vi "Watchdog (SubVI).vi"(7 "System Message Queue In":refnum<queue>, 8 "error in (no error)":errorcluster, 11 "Enable Watchdog?":bool) -> (0 "error out":errorcluster)   [LabVIEW 2019]
uses:
  Globals and Definitions/System Message.ctl
  <vilib>/RTwatchdog.llb/Watchdog expiration actions.ctl
  <vilib>/RTwatchdog.llb/Watchdog status enum.ctl
  Globals and Definitions/Initialization Globals.vi
  Globals and Definitions/RT Globals RD v1.0.vi
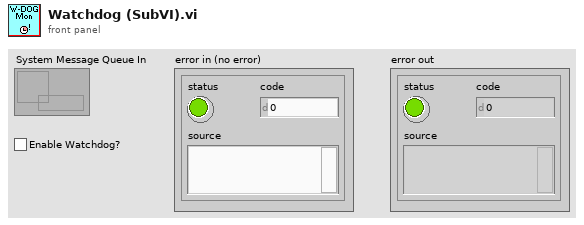
[diagram p1: front panel]
types:
  T1 = typedef "System Message.ctl" = cluster{"Message Tag":string, "Message Body":string, "Snooze Time (s)":dbl, "Snooze Alert?":bool, "Log Event?":bool, "Send Email":i32}
  T2 = typedef "Watchdog expiration actions.ctl" = cluster{"reset system":bool, "restart LabVIEW Runtime":bool, "occurrence":bool, "trigger protocol":enum16{"active high", "active low", "open collector"}, "trigger line":enum16{"none", "line 0", "line 1", "line 2", "line 3", "line 4", "line 5", "line 6", "line 7", "SMB line 0"}, "disable watchdog on VI exit":bool}
  T3 = typedef "Watchdog status enum.ctl" = enum16{"disabled", "expired", "running"}
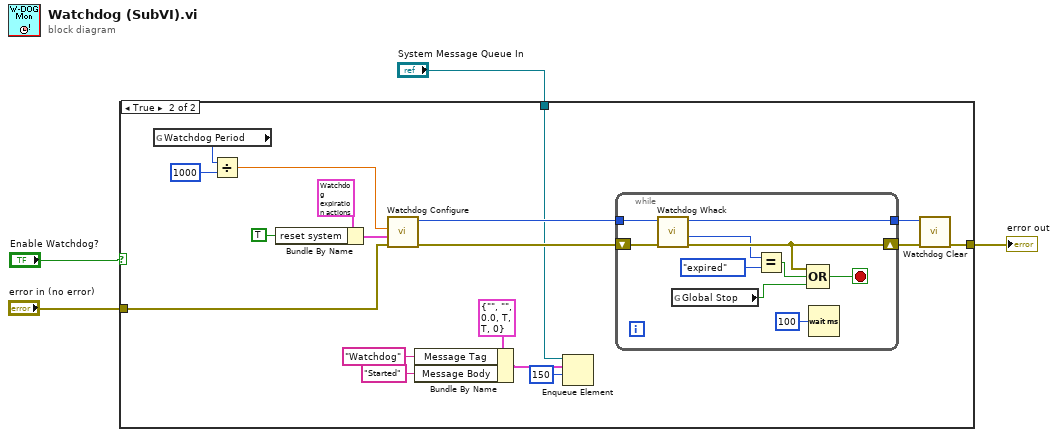
[diagram p0: block diagram]
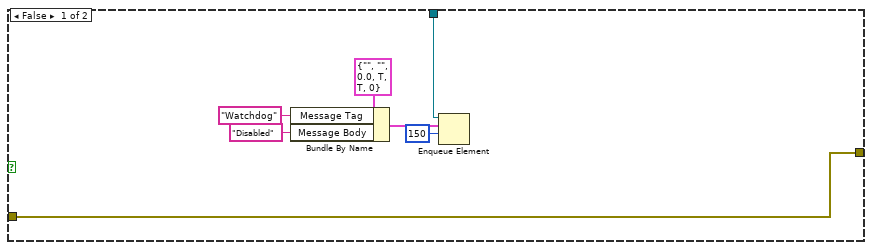
[diagram p2: hidden frame]
diagram:
  n1 = case shown="True" "Enable Watchdog?" {
    tunnel: "error in (no error)" -> [w11 w23]
    tunnel: [w11 w22] -> w2
    tunnel: "System Message Queue In" -> [w6 w15]
    frame False {
      n2 = Bundle By Name(cluster=T1 {"Message Tag"="", "Message Body"="", "Snooze Time (s)"=0.0, "Snooze Alert?"=TRUE, "Log Event?"=TRUE, "Send Email"=0}, "Message Tag"="Watchdog", "Message Body"="Disabled") -> (w5:T1)
      n3 = Enqueue Element(queue=w6, element=w5, timeout in ms (-1)=150) -> ()  [unwired: 1 in, 3 out]
    }
    frame True {
      n4 = global read "Initialization Globals.vi" "Watchdog Period"() -> (w21:u32)
      n5 = Divide(x=w21, y=u32 1000) -> (x/y=w19:dbl)
      n6 = Bundle By Name(cluster=T2 {"reset system"=FALSE, "restart LabVIEW Runtime"=FALSE, "occurrence"=FALSE, "trigger protocol"=enum."active high", "trigger line"=enum."none", "disable watchdog on VI exit"=TRUE} ("expiration actions"), "reset system"=TRUE) -> (w28:T2)
      n7 = call <vilib>:"Watchdog Configure.vi"("error in (no error)"=w23, "expiration actions"=w28, "timeout (1 sec)"=w19) -> ("error out"=w26:errorcluster, "watchdogID"=w27:u64)  [unwired: 1 in, 2 out]
      n8 = Bundle By Name(cluster=T1 {"Message Tag"="", "Message Body"="", "Snooze Time (s)"=0.0, "Snooze Alert?"=TRUE, "Log Event?"=TRUE, "Send Email"=0}, "Message Tag"="Watchdog", "Message Body"="Started") -> (w17:T1)
      n9 = Enqueue Element(queue=w15, element=w17, timeout in ms (-1)=150) -> ()  [unwired: 1 in, 3 out]
      n10 = while {
        tunnel: [w37] -> w25
        tunnel: w27 -> [w38]
        shift-right: [w35] -> w24
        shift-left: w26 -> [w39]
        stop <- w36 stop-if-true
        n11 = call <vilib>:"Watchdog Whack.vi"("error in (no error)"=w39, "watchdogID in"=w38) -> ("error out"=w35:errorcluster, "watchdog status"=w34:T3, "watchdogID out"=w37:u64)  [unwired: 3 in]
        n12 = global read "RT Globals RD v1.0.vi" "Global Stop"() -> (w31:bool)
        n13 = Equal?(x=w34, y=Watchdog_status_enum."expired") -> (x = y?=w32:bool)
        n14 = Compound Arithmetic op=OR(w35, w32, w31) -> (w36:bool)
        n15 = Wait (ms)(milliseconds to wait=u32 100) -> ()  [unwired: 1 out]
      }
      n16 = call <vilib>:"Watchdog Clear.vi"("error in (no error)"=w24, "watchdogID in"=w25) -> ("error out"=w22:errorcluster)  [unwired: 5 in]
    }
  }
  "error out" <- w2
